vi "DriveTrainCals.vi"() -> ()   [LabVIEW 2014]
panel:
  in  "CorrectWithinXDegrees":dbl
  in  "YawProportionalFeedback":dbl=0.005
  in  "TurnEpsilon":dbl=0.1
  in  "MaxUltraSonic":dbl=3.0
  in  "MinUltraSonic":dbl=0.3
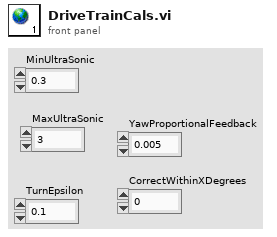
[diagram p1: front panel]
diagram:
